vi "SendEventRefRoutedMessage_Name.vi"() -> (1 "message name":string)   [LabVIEW 2017, in "FileManager.lvlib"]
uses:
  <vilib>/addons/InsightCM/Devices/Shared/Common/FileManager/FileManager.lvlib
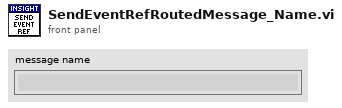
[diagram p1: front panel]
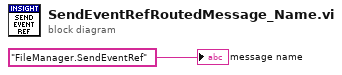
[diagram p0: block diagram]
diagram:
  "message name" <- "FileManager.SendEventRef" ("ProcessName")
